vi "addOutcome.vi"(8 "error in (no error)":errorcluster, 10 "Outcome.lvclass":refnum<class "Outcome.lvclass">, 11 "OutcomeList in":refnum<class "OutcomeList.lvclass">) -> (0 "error out":errorcluster, 3 "OutcomeList out":refnum<class "OutcomeList.lvclass">)   [LabVIEW 2018, in "OutcomeList.lvclass"]
uses:
  OutcomeList.lvclass
  Expense Summary/Outcome.lvclass
  OutcomeList.lvclass/OutcomeList.ctl
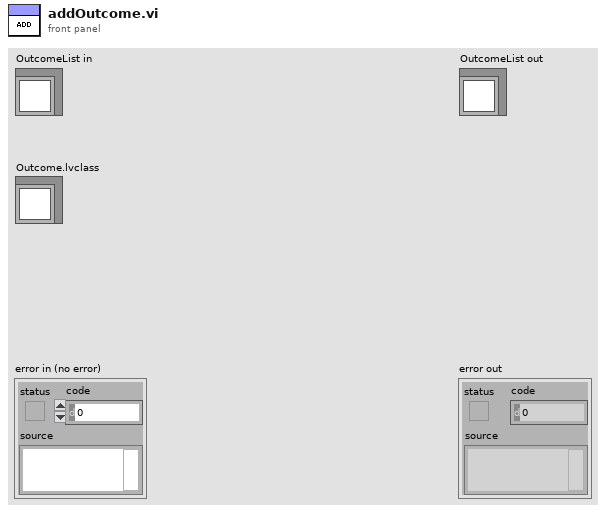
[diagram p1: front panel]
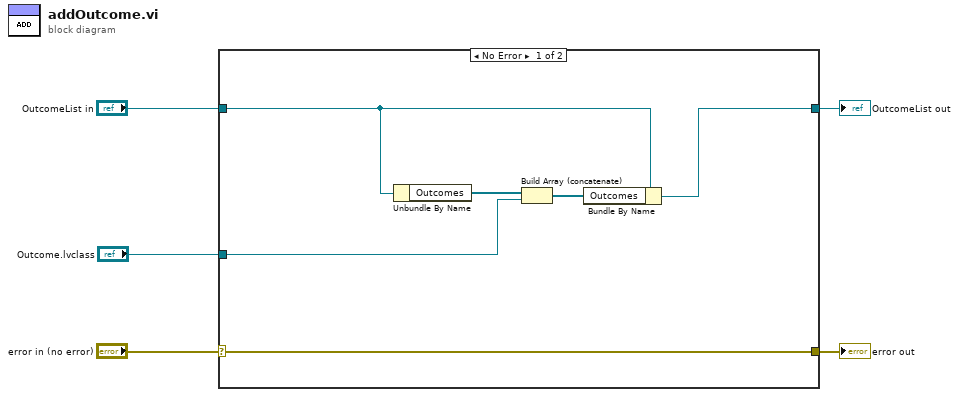
[diagram p0: block diagram]
diagram:
  n1 = case shown="No Error" "error in (no error)" {
    selector: "error in (no error)" -> [w11 w13]
    tunnel: [w11 w13] -> w4
    tunnel: [w9 w12] -> w2
    tunnel: "OutcomeList in" -> [w10 w12]
    tunnel: "Outcome.lvclass" -> [w7 _]
    frame No Error {
      n2 = Unbundle By Name(w10) -> ("Outcomes"=w8:refnum<class "Outcome.lvclass">[])
      n3 = Build Array (concatenate)(w8, w7) -> (w6:refnum<class "Outcome.lvclass">[])
      n4 = Bundle By Name(cluster=w10, "Outcomes"=w6) -> (w9:refnum<class "OutcomeList.lvclass">)
    }
    frame Error {
    }
  }
  "error out" <- w4
  "OutcomeList out" <- w2
